vi "Write auto error handling.vi"(8 "error in (no error)":errorcluster, 10 "auto error handling":bool, 11 "execution settings in":refnum<class "execution settings.lvclass">) -> (0 "error out":errorcluster, 3 "execution settings out":refnum<class "execution settings.lvclass">)   [LabVIEW 2013, in "execution settings.lvclass"]
uses:
  execution settings.lvclass
  execution settings.lvclass/execution settings.ctl
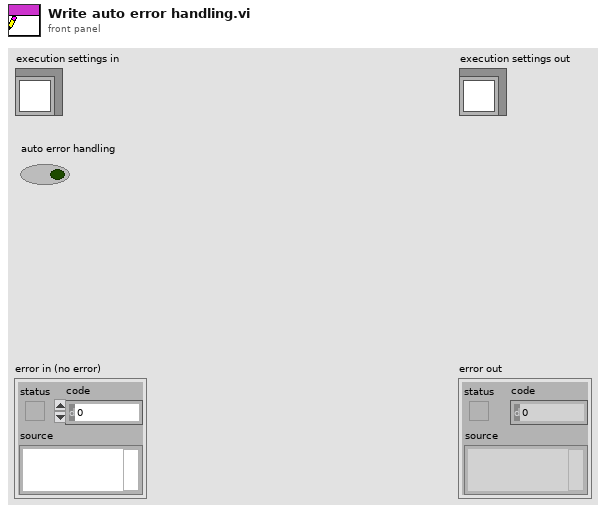
[diagram p1: front panel]
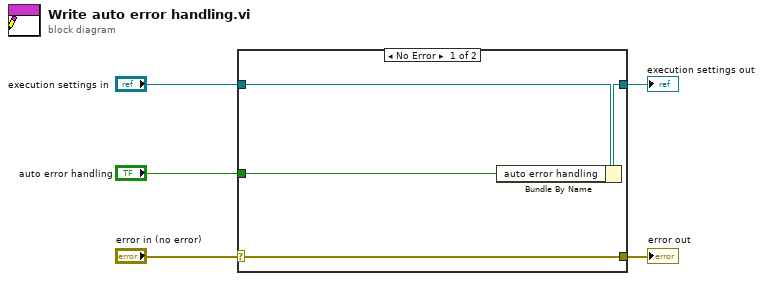
[diagram p0: block diagram]
diagram:
  n1 = case shown="No Error" "error in (no error)" {
    selector: "error in (no error)" -> [w9 w10]
    tunnel: [w9 w10] -> w4
    tunnel: [w7 w11] -> w2
    tunnel: "execution settings in" -> [w8 w11]
    tunnel: "auto error handling" -> [w6 _]
    frame No Error {
      n2 = Bundle By Name(cluster=w8, "auto error handling"=w6) -> (w7:refnum<class "execution settings.lvclass">)
    }
    frame Error {
    }
  }
  "error out" <- w4
  "execution settings out" <- w2
